vi "UI_Test_Template_Manage.vi"() -> ()   [LabVIEW 2014]
uses:
  Terminal_Global_Template_Name.vi
panel:
  out "载荷谱列表":string[][](table)
  in  "退出":bool
  # "载荷谱模板维护"
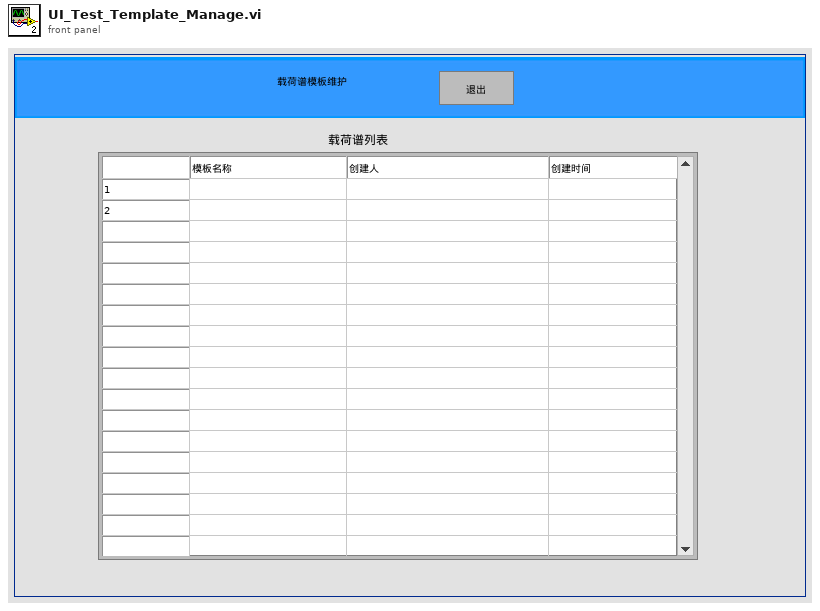
[diagram p1: front panel]
types:
  T1 = typedef "LVPoint32TypeDef.ctl" = cluster{"Horizontal":i32, "Vertical":i32}
  T2 = typedef "LVRowAndColumnTypeDef.ctl" = cluster{"Row":i32, "Column":i32}
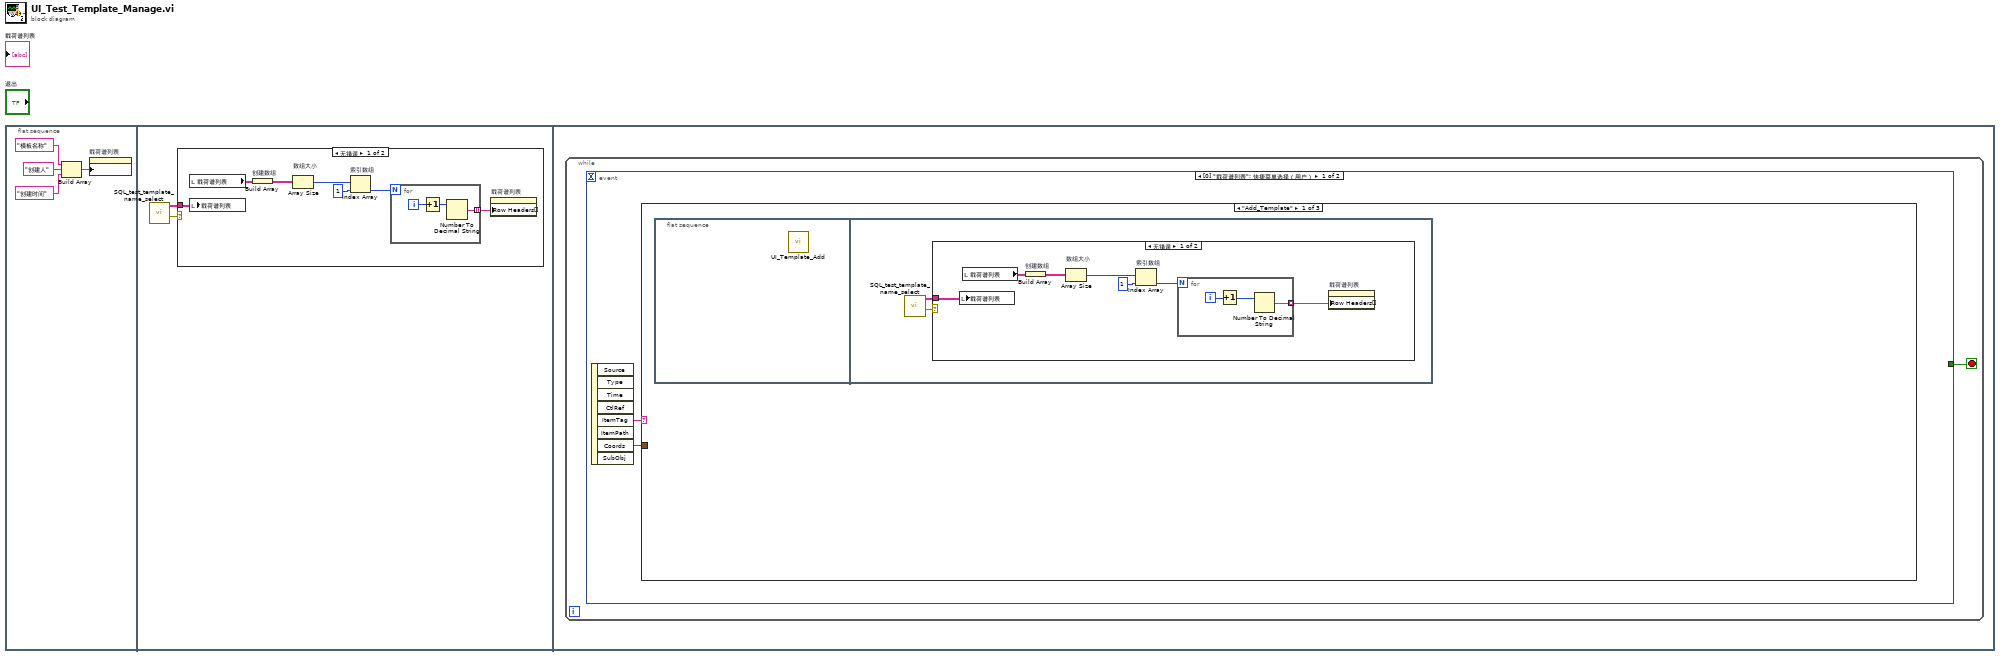
[diagram p0: block diagram]
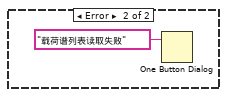
[diagram p2: hidden frame]
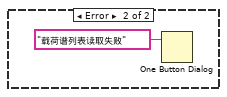
[diagram p3: hidden frame]
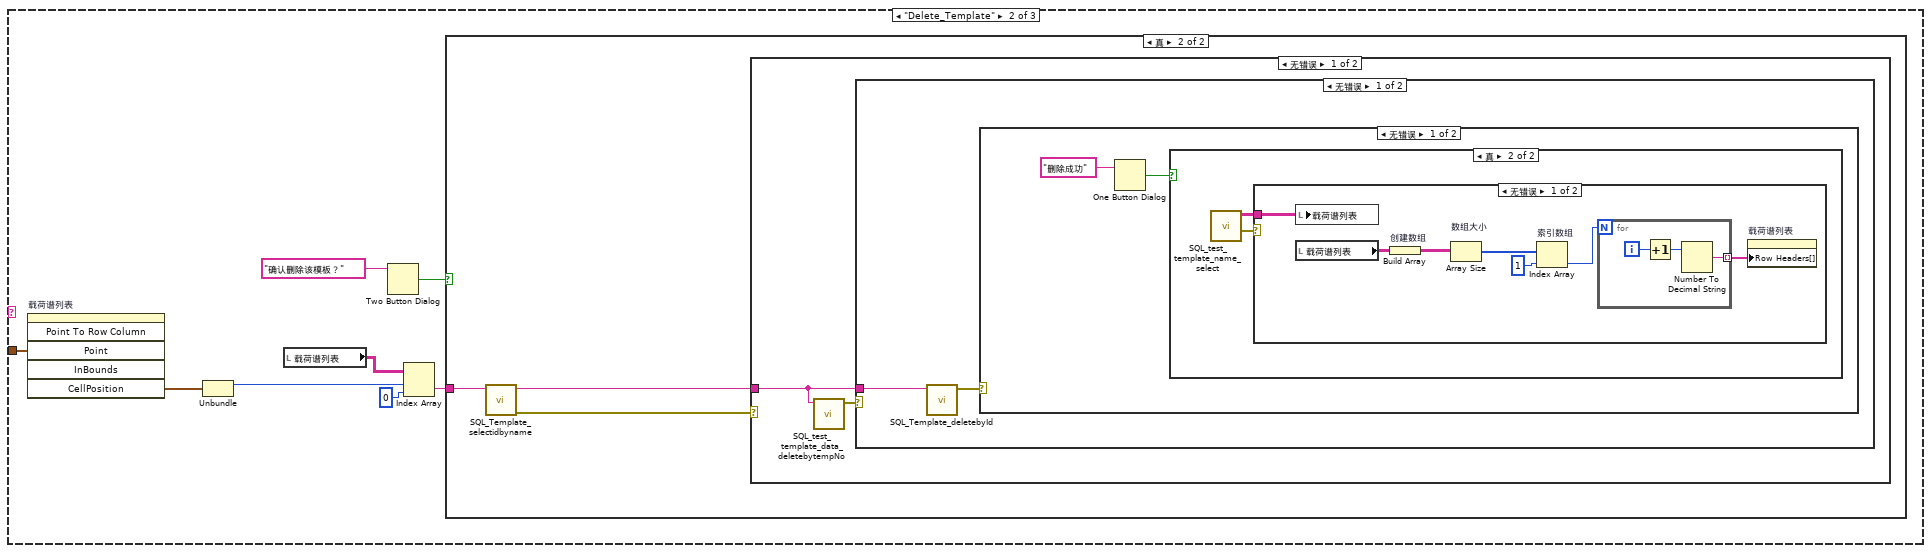
[diagram p4: hidden frame]
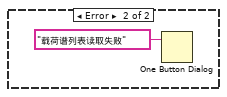
[diagram p7: hidden frame]
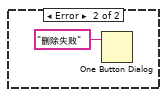
[diagram p9: hidden frame]
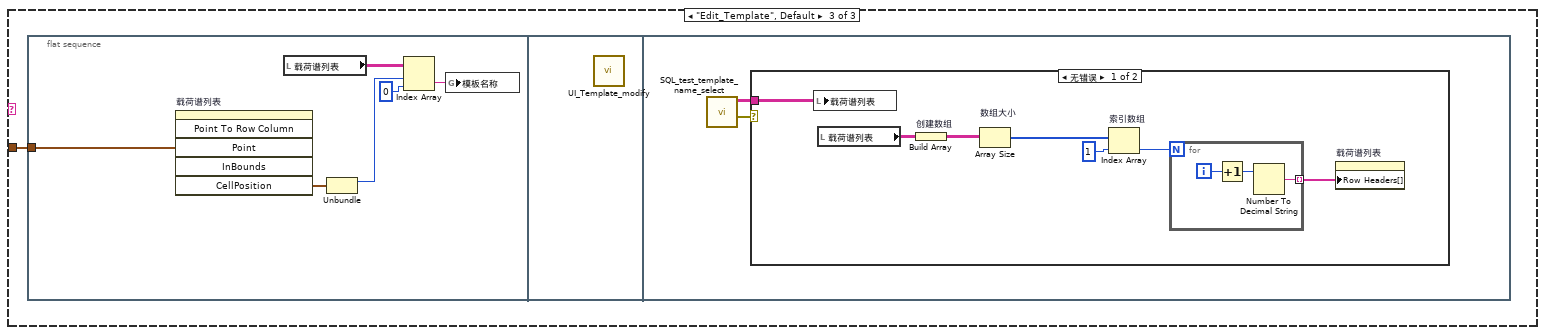
[diagram p11: hidden frame]
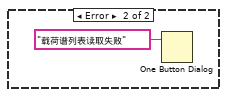
[diagram p12: hidden frame]
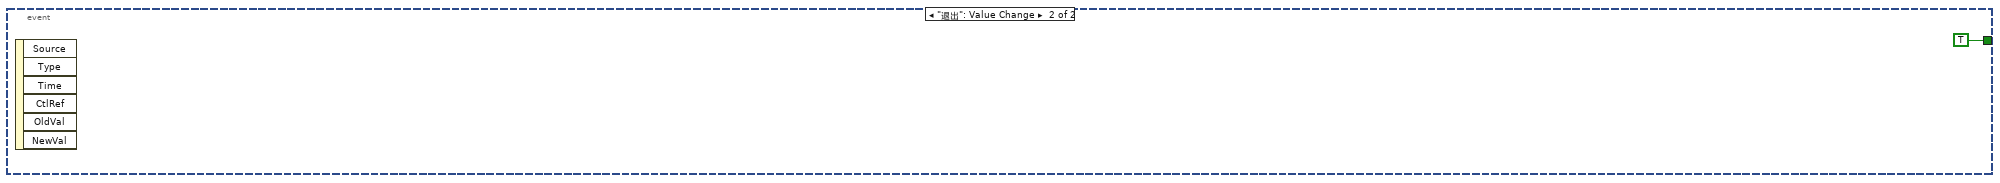
[diagram p13: hidden frame]
diagram:
  n1 = flat-sequence {
    frame #0 {
      n2 = Build Array("模板名称", "创建人", "创建时间") -> (w1:string[])
      n3 = property on="载荷谱列表" class="Tbl (严格)"("Column Headers[]"=w1) -> ()  [unwired: 2 in, 2 out]
    }
    frame #1 {
      n4 = call "SQL_test_template_name_select.vi"() -> ("error out"=w6:errorcluster, "模板名称"=w5:string[][])  [unwired: 10 in]
      n5 = case shown="无错误" w6 {
        tunnel: w5 -> [w7 _]
        frame No Error {
          n6 = local read "载荷谱列表"() -> (w10:string[][])
          n7 = local write "载荷谱列表"(w7) -> ()
          n8 = Build Array "创建数组"(w10) -> (w11:string[][][])
          n9 = Array Size "数组大小"(array=w11) -> (size(s)=w12:i32[])
          n10 = Index Array "索引数组"(array=w12, index=1) -> (element=w8:i32)
          n11 = for {
            N: w8 -> [_]
            tunnel: [w16] -> w9 mode=indexing
            i -> [w15]
            n12 = Increment(x=w15) -> (x+1=w14:i32)
            n13 = Number To Decimal String(number=w14) -> (decimal integer string=w16:string)  [unwired: 1 in]
          }
          n14 = property on="载荷谱列表" class="Tbl (严格)"("Row Headers[]"=w9) -> ()  [unwired: 2 in, 2 out]
        }
        frame Error {
          n15 = One Button Dialog(message="载荷谱列表读取失败" ("消息")) -> ()  [unwired: 1 in, 1 out]
        }
      }
    }
    frame #2 {
      n16 = while {
        stop <- w18 stop-if-true
        n17 = event shown="[0] \"载荷谱列表\": 快捷菜单选择（用户）" {
          selector: _ -> [_ _]
          dyn-events: _ -> [_ _]
          timeout: _ -> [_ _]
          tunnel: [_ TRUE] -> w18
          event "载荷谱列表": Shortcut Menu Selection (User) {
            n18 = event-data() -> ("ItemTag"=w20:string, "Coords"=w19:T1)  [unwired: 1 in, 6 out]
            n19 = case shown="\"Add_Template\"" w20 {
              tunnel: w19 -> [_ w40 w65]
              frame "Add_Template" {
                n20 = flat-sequence {
                  frame #0 {
                    n21 = call "UI_Template_Add.vi"() -> ()  [unwired: 12 in]
                  }
                  frame #1 {
                    n22 = call "SQL_test_template_name_select.vi"() -> ("error out"=w22:errorcluster, "模板名称"=w21:string[][])  [unwired: 10 in]
                    n23 = case shown="无错误" w22 {
                      tunnel: w21 -> [w24 _]
                      frame No Error {
                        n24 = local write "载荷谱列表"(w24) -> ()
                        n25 = local read "载荷谱列表"() -> (w26:string[][])
                        n26 = Build Array "创建数组"(w26) -> (w27:string[][][])
                        n27 = Array Size "数组大小"(array=w27) -> (size(s)=w28:i32[])
                        n28 = Index Array "索引数组"(array=w28, index=1) -> (element=w25:i32)
                        n29 = for {
                          N: w25 -> [_]
                          tunnel: [w32] -> w23 mode=indexing
                          i -> [w31]
                          n30 = Increment(x=w31) -> (x+1=w30:i32)
                          n31 = Number To Decimal String(number=w30) -> (decimal integer string=w32:string)  [unwired: 1 in]
                        }
                        n32 = property on="载荷谱列表" class="Tbl (严格)"("Row Headers[]"=w23) -> ()  [unwired: 2 in, 2 out]
                      }
                      frame Error {
                        n33 = One Button Dialog(message="载荷谱列表读取失败" ("消息")) -> ()  [unwired: 1 in, 1 out]
                      }
                    }
                  }
                }
              }
              frame "Delete_Template" {
                n34 = invoke on="载荷谱列表" class="Tbl (严格)" method="Point To Row Column"("Point"=w40) -> ("CellPosition"=w39:T2)  [unwired: 5 in, 5 out]
                n35 = Unbundle(w39) -> ("Row"=w36:i32)  [unwired: 1 out]
                n36 = local read "载荷谱列表"() -> (w37:string[][])
                n37 = Two Button Dialog(message="确认删除该模板？" ("消息")) -> (T button?=w38:bool)  [unwired: 2 in]
                n38 = Index Array(array=w37, index (row)=w36, index (col)=0 ("禁用的索引 (列)")) -> (element=w34:string)
                n39 = case shown="真" w38 {
                  tunnel: w34 -> [_ w44]
                  frame False {
                  }
                  frame True {
                    n40 = call "SQL_Template_selectidbyname.vi"("模板名称"=w44) -> ("error out"=w42:errorcluster, "tempNo"=w43:string)  [unwired: 9 in]
                    n41 = case shown="无错误" w42 {
                      tunnel: w43 -> [w45 _]
                      frame No Error {
                        n42 = call "SQL_test_template_data_deletebytempNo.vi"("tempNo"=w45) -> ("error out"=w46:errorcluster)  [unwired: 10 in]
                        n43 = case shown="无错误" w46 {
                          tunnel: w45 -> [w48 _]
                          frame No Error {
                            n44 = call "SQL_Template_deletebyId.vi"("tempNo"=w48) -> ("error out"=w47:errorcluster)  [unwired: 10 in]
                            n45 = case shown="无错误" w47 {
                              frame No Error {
                                n46 = One Button Dialog(message="删除成功" ("消息")) -> (true=w49:bool)  [unwired: 1 in]
                                n47 = case shown="真" w49 {
                                frame False {
                                }
                                frame True {
                                n48 = call "SQL_test_template_name_select.vi"() -> ("error out"=w52:errorcluster, "模板名称"=w51:string[][])  [unwired: 10 in]
                                n49 = case shown="无错误" w52 {
                                tunnel: w51 -> [w54 _]
                                frame No Error {
                                n50 = local write "载荷谱列表"(w54) -> ()
                                n51 = local read "载荷谱列表"() -> (w56:string[][])
                                n52 = Build Array "创建数组"(w56) -> (w57:string[][][])
                                n53 = Array Size "数组大小"(array=w57) -> (size(s)=w58:i32[])
                                n54 = Index Array "索引数组"(array=w58, index=1) -> (element=w55:i32)
                                n55 = for {
                                N: w55 -> [_]
                                tunnel: [w62] -> w53 mode=indexing
                                i -> [w61]
                                n56 = Increment(x=w61) -> (x+1=w60:i32)
                                n57 = Number To Decimal String(number=w60) -> (decimal integer string=w62:string)  [unwired: 1 in]
                                }
                                n58 = property on="载荷谱列表" class="Tbl (严格)"("Row Headers[]"=w53) -> ()  [unwired: 2 in, 2 out]
                                }
                                frame Error {
                                n59 = One Button Dialog(message="载荷谱列表读取失败" ("消息")) -> ()  [unwired: 1 in, 1 out]
                                }
                                }
                                }
                                }
                              }
                              frame Error {
                              }
                            }
                          }
                          frame Error {
                            n60 = One Button Dialog(message="删除失败" ("消息")) -> ()  [unwired: 1 in, 1 out]
                          }
                        }
                      }
                      frame Error {
                      }
                    }
                  }
                }
              }
              frame "Edit_Template", Default {
                n61 = flat-sequence {
                  tunnel: w65 -> [w71]
                  frame #0 {
                    n62 = invoke on="载荷谱列表" class="Tbl (严格)" method="Point To Row Column"("Point"=w71) -> ("CellPosition"=w70:T2)  [unwired: 5 in, 5 out]
                    n63 = local read "载荷谱列表"() -> (w69:string[][])
                    n64 = Unbundle(w70) -> ("Row"=w68:i32)  [unwired: 1 out]
                    n65 = Index Array(array=w69, index (row)=w68, index (col)=0 ("禁用的索引 (列)")) -> (element=w66:string)
                    n66 = global write "Terminal_Global_Template_Name.vi" "模板名称"(w66) -> ()
                  }
                  frame #1 {
                    n67 = call "UI_Template_modify.vi"() -> ()  [unwired: 12 in]
                  }
                  frame #2 {
                    n68 = call "SQL_test_template_name_select.vi"() -> ("error out"=w73:errorcluster, "模板名称"=w72:string[][])  [unwired: 10 in]
                    n69 = case shown="无错误" w73 {
                      tunnel: w72 -> [w75 _]
                      frame No Error {
                        n70 = local write "载荷谱列表"(w75) -> ()
                        n71 = local read "载荷谱列表"() -> (w77:string[][])
                        n72 = Build Array "创建数组"(w77) -> (w78:string[][][])
                        n73 = Array Size "数组大小"(array=w78) -> (size(s)=w79:i32[])
                        n74 = Index Array "索引数组"(array=w79, index=1) -> (element=w76:i32)
                        n75 = for {
                          N: w76 -> [_]
                          tunnel: [w83] -> w74 mode=indexing
                          i -> [w82]
                          n76 = Increment(x=w82) -> (x+1=w81:i32)
                          n77 = Number To Decimal String(number=w81) -> (decimal integer string=w83:string)  [unwired: 1 in]
                        }
                        n78 = property on="载荷谱列表" class="Tbl (严格)"("Row Headers[]"=w74) -> ()  [unwired: 2 in, 2 out]
                      }
                      frame Error {
                        n79 = One Button Dialog(message="载荷谱列表读取失败" ("消息")) -> ()  [unwired: 1 in, 1 out]
                      }
                    }
                  }
                }
              }
            }
          }
          event "退出": Value Change {
            n80 = event-data() -> ()  [unwired: 1 in, 6 out]
          }
        }
      }
    }
  }
